vi "Get Class Methods from ClassName.vi"(0 "App Ref":refnum<vi>, 1 "Class Name":string, 3 "error in":errorcluster) -> (4 "Access Scopes":T1(array[ring]), 5 "Wire Pens":T2(array[cluster]), 6 "dup App Ref":refnum<vi>, 7 "Method Names":string[](array[string]), 8 "Method VIs":refnum<vi>[](array[refnum]), 9 "error out":errorcluster)   [LabVIEW 2025, in "XNode Support.lvlib"]
uses:
  XNode Support.lvlib
  <vilib>/regexp/Match Regular Expression.xnode
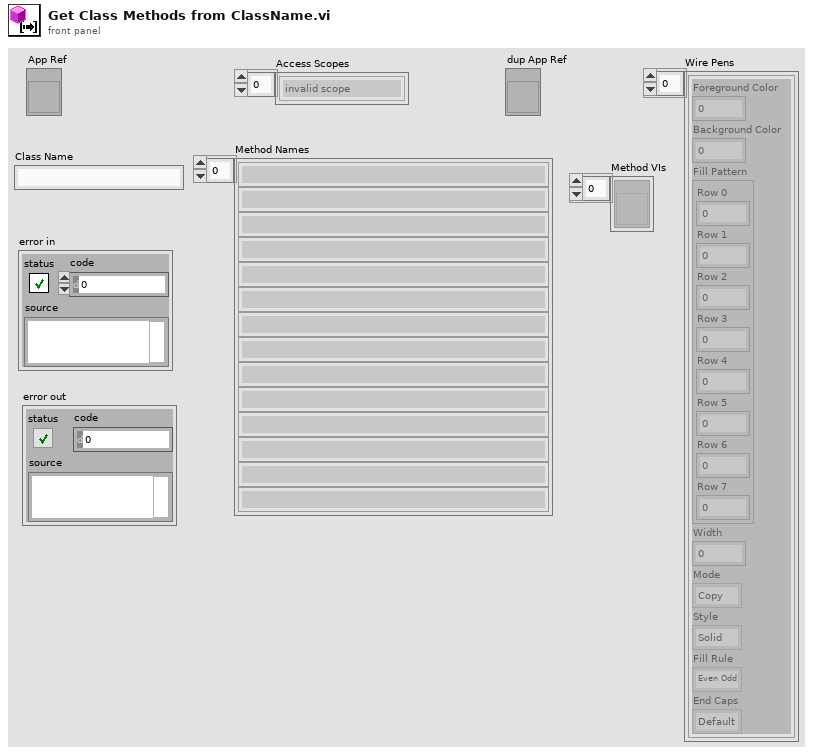
[diagram p1: front panel]
types:
  T1 = enum32{"invalid scope", "public", "private", "protected", "community"}[]
  T2 = cluster{"Foreground Color":u32, "Background Color":u32, "Fill Pattern":cluster{"Row 0":u8, "Row 1":u8, "Row 2":u8, "Row 3":u8, "Row 4":u8, "Row 5":u8, "Row 6":u8, "Row 7":u8}, "Width":i16, "Mode":enum16{"Copy", "Or", "Exclusive Or", "Bit Clear", "Not Copy", "Not Or", "Nor Exclusive Or", "Not Bit Clear"}, "Style":enum32{"Solid", "Dash", "Dot", "Dash Dot", "Dash Dot Dot"}, "Fill Rule":enum32{"Even Odd", "Winding"}, "End Caps":enum32{"Default", "Flat"}}[]
  T3 = enum32{"invalid scope", "public", "private", "protected", "community"}
  T4 = enum32{"invalid VI type", "Standard VI", "Control VI", "Global VI", "Polymorphic VI", "Configuration VI", "SubSystem", "Facade VI", "Method VI", "Statechart Diagram VI"}
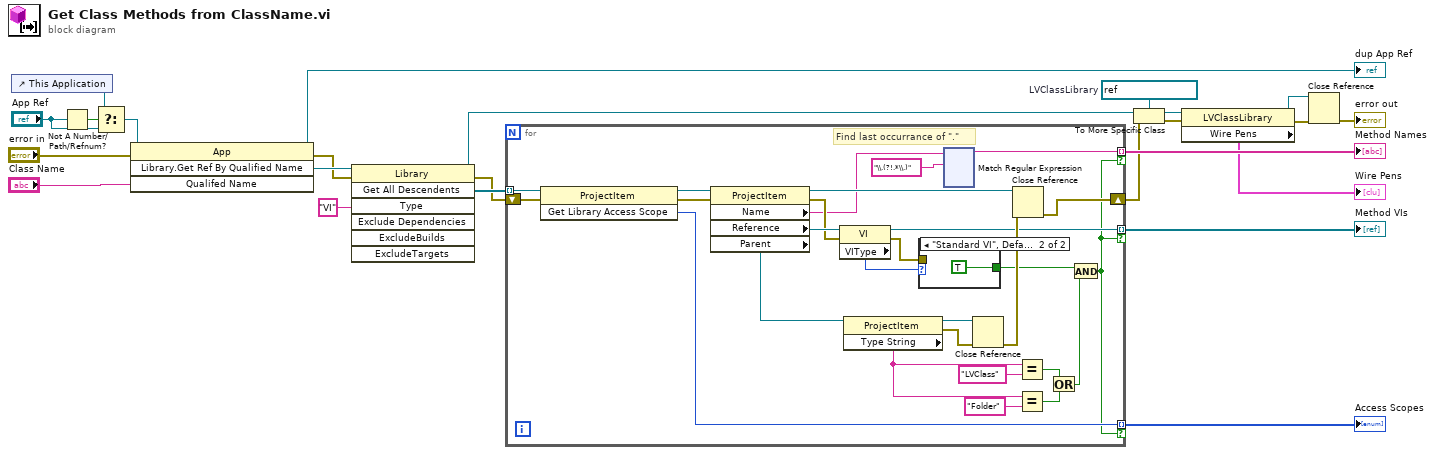
[diagram p0: block diagram]
diagram:
  w8 = refnum<vi> refnum  # LVClassLibrary
  n1 = control-ref of="This Application"() -> (w15:refnum<vi>)
  n2 = Not A Number/Path/Refnum?(number/path/refnum="App Ref") -> (NaN/Path/Refnum?=w14:bool)
  n3 = Select(t=w15, s=w14, f="App Ref") -> (s? t:f=w12:refnum<vi>)
  n4 = invoke class="App" method="Library.Get Ref By Qualified Name"(reference=w12, error in="error in", "Qualifed Name"="Class Name") -> (reference out=→"dup App Ref":refnum<vi>, error out=w19:errorcluster, "Library.Get Ref By Qualified Name"=w23:refnum<vi>)  [unwired: 1 in, 1 out]
  n5 = invoke class="Library" method="Get All Descendents"(reference=w23, error in=w19, "Type"="VI") -> (reference out=w10:refnum<vi>, error out=w20:errorcluster, "All Descendents"=w24:refnum<vi>[])  [unwired: 4 in, 4 out]
  n6 = for {
    tunnel: w24 -> [w51] mode=indexing
    tunnel: [w42] -> w21 mode=indexing if=w28
    tunnel: [w26] -> w22 mode=indexing if=w28
    shift-right: [w44] -> w9
    shift-left: w20 -> [w31]
    tunnel: [w29] -> w1 mode=indexing if=w28
    # "Find last occurrance of \".\""
    n7 = invoke class="ProjectItem" method="Get Library Access Scope"(reference=w51, error in=w31) -> (reference out=w32:refnum<vi>, error out=w30:errorcluster, "Get Library Access Scope"=w29:T3)  [unwired: 1 in]
    n8 = property class="ProjectItem"(reference=w32, error in=w30) -> (reference out=w46:refnum<vi>, error out=w41:errorcluster, "Name"=w27:string, "Reference"=w43:refnum<vi>, "Parent"=w50:refnum<vi>)
    n9 = property class="VI"(reference=w43, error in=w41) -> (reference out=w42:refnum<vi>, error out=w38:errorcluster, "VIType"=w40:T4)
    n10 = property class="ProjectItem"(reference=w50) -> (reference out=w48:refnum<vi>, error out=w47:errorcluster, "Type String"=w36:string)  [unwired: 1 in]
    n11 = case shown="\"Standard VI\", Default" w40 {
      tunnel: [_ TRUE] -> w39
      tunnel: w38 -> [_ _]
      frame "invalid VI type", "Control VI", "Global VI" {
      }
      frame "Standard VI", Default {
      }
    }
    n12 = xnode "Match Regular Expression"("input string"=w27, "regular expression"="\\.(?!.*\\.)") -> ("before match"=w26:string)  [unwired: 4 in, 4 out]
    n13 = Close Reference(reference=w48, error in (no error)=w47) -> (error out=w45:errorcluster)
    n14 = Close Reference(reference=w46, error in (no error)=w45) -> (error out=w44:errorcluster)
    n15 = Equal?(x=w36, y="LVClass") -> (x = y?=w34:bool)
    n16 = Equal?(x=w36, y="Folder") -> (x = y?=w35:bool)
    n17 = Or(x=w34, y=w35) -> (x .or. y?=w33:bool)
    n18 = And(x=w39, y=w33) -> (x .and. y?=w28:bool)
  }
  "Method Names" <- w22
  "Method VIs" <- w21
  "Access Scopes" <- w1
  n19 = To More Specific Class(target class=w8, reference=w10, error in=w9) -> (specific class reference=w7:refnum<vi>, error out=w6:errorcluster)
  n20 = property class="LVClassLibrary"(reference=w7, error in=w6) -> (reference out=w3:refnum<vi>, error out=w4:errorcluster, "Wire Pens"=→"Wire Pens":T2)
  n21 = Close Reference(reference=w3, error in (no error)=w4) -> (error out=→"error out":errorcluster)
